vi "Control Scaling.vi"(1 "Position to go":T1={"X"=FALSE, "Target X (um)"=1000.0, "Current X (um)"=1000.0, "Scaling X"=0, "Y"=FALSE, "Target Y (um)"=0.0, "Current Y (um)"=0.0, "Scaling Y"=0, "Z"=FALSE, "Target Z (um)"=0.0, "Current Z (um)"=0.0, "Scaling Z"=0} {"Current X (um)" step=1.0; "Scaling Z" items=["X", "Z", "None"]; "Scaling Y" items=["X", "Z", "None"]; "Scaling X" items=["X", "Z", "None"]; "Target X (um)" step=1.0}) -> (0 "Position to go out":T2)   [LabVIEW 2014]
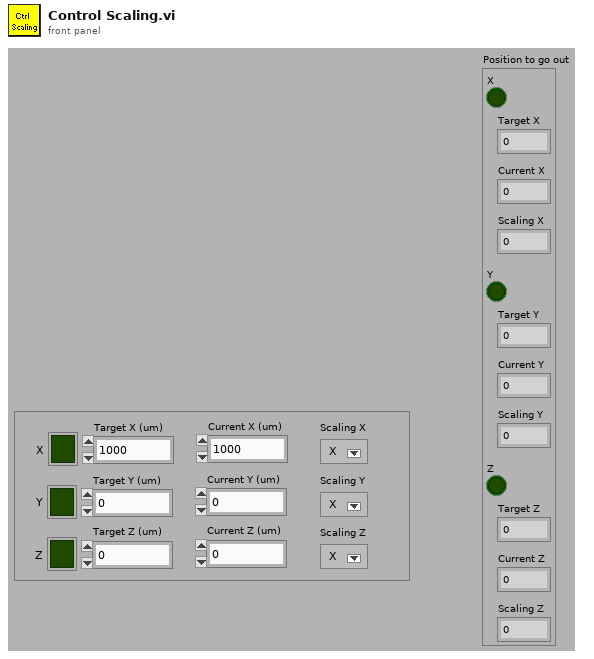
[diagram p1: front panel]
types:
  T1 = cluster{"X":bool, "Target X (um)":dbl, "Current X (um)":dbl, "Scaling X":u16, "Y":bool, "Target Y (um)":dbl, "Current Y (um)":dbl, "Scaling Y":u16, "Z":bool, "Target Z (um)":dbl, "Current Z (um)":dbl, "Scaling Z":u16}
  T2 = cluster{"X":bool, "Target X ":dbl, "Current X":dbl, "Scaling X":u16, "Y":bool, "Target Y":dbl, "Current Y":dbl, "Scaling Y":u16, "Z":bool, "Target Z":dbl, "Current Z":dbl, "Scaling Z":u16}
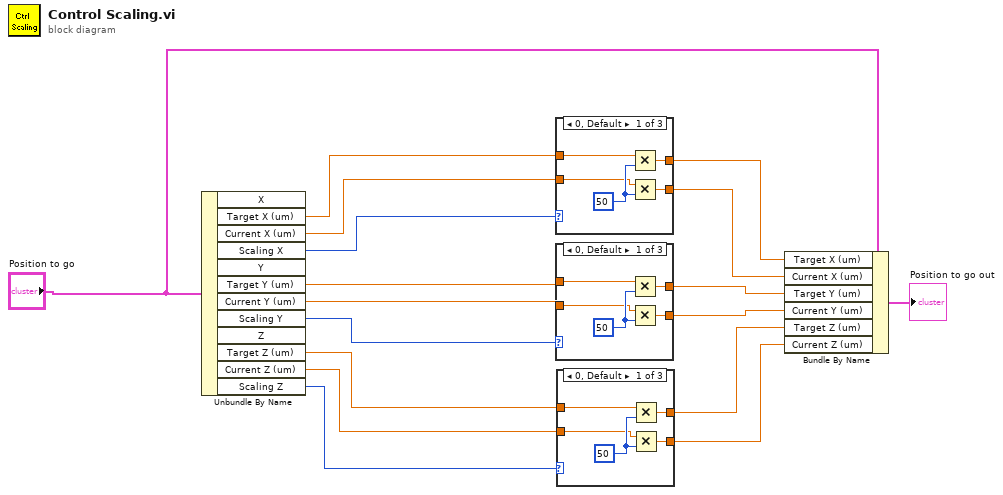
[diagram p0: block diagram]
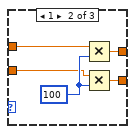
[diagram p2: hidden frame]
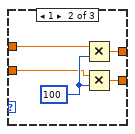
[diagram p4: hidden frame]
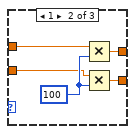
[diagram p6: hidden frame]
diagram:
  n1 = Unbundle By Name("Position to go") -> ("Target X (um)"=w17:dbl, "Current X (um)"=w16:dbl, "Scaling X"=w15:u16, "Target Y (um)"=w14:dbl, "Current Y (um)"=w13:dbl, "Scaling Y"=w12:u16, "Target Z (um)"=w10:dbl, "Current Z (um)"=w9:dbl, "Scaling Z"=w11:u16)  [unwired: 3 out]
  n2 = case shown="0, Default" w15 {
    tunnel: [w22 w25 w28] -> w7
    tunnel: w17 -> [w20 w24 w29]
    tunnel: w16 -> [w19 w23 w28]
    tunnel: [w18 w26 w29] -> w8
    frame 0, Default {
      w21 = 50
      n3 = Multiply(x=w20, y=w21) -> (x*y=w18:dbl)
      n4 = Multiply(x=w19, y=w21) -> (x*y=w22:dbl)
    }
    frame 1 {
      w27 = 100
      n5 = Multiply(x=w24, y=w27) -> (x*y=w26:dbl)
      n6 = Multiply(x=w23, y=w27) -> (x*y=w25:dbl)
    }
    frame 2 {
    }
  }
  n7 = case shown="0, Default" w12 {
    tunnel: [w34 w37 w40] -> w5
    tunnel: w14 -> [w32 w36 w41]
    tunnel: w13 -> [w31 w35 w40]
    tunnel: [w30 w38 w41] -> w6
    frame 0, Default {
      w33 = 50
      n8 = Multiply(x=w32, y=w33) -> (x*y=w30:dbl)
      n9 = Multiply(x=w31, y=w33) -> (x*y=w34:dbl)
    }
    frame 1 {
      w39 = 100
      n10 = Multiply(x=w36, y=w39) -> (x*y=w38:dbl)
      n11 = Multiply(x=w35, y=w39) -> (x*y=w37:dbl)
    }
    frame 2 {
    }
  }
  n12 = case shown="0, Default" w11 {
    tunnel: [w46 w49 w52] -> w3
    tunnel: w10 -> [w44 w48 w53]
    tunnel: w9 -> [w43 w47 w52]
    tunnel: [w42 w50 w53] -> w4
    frame 0, Default {
      w45 = 50
      n13 = Multiply(x=w44, y=w45) -> (x*y=w42:dbl)
      n14 = Multiply(x=w43, y=w45) -> (x*y=w46:dbl)
    }
    frame 1 {
      w51 = 100
      n15 = Multiply(x=w48, y=w51) -> (x*y=w50:dbl)
      n16 = Multiply(x=w47, y=w51) -> (x*y=w49:dbl)
    }
    frame 2 {
    }
  }
  n17 = Bundle By Name(cluster="Position to go", "Target X (um)"=w8, "Current X (um)"=w7, "Target Y (um)"=w6, "Current Y (um)"=w5, "Target Z (um)"=w4, "Current Z (um)"=w3) -> (→"Position to go out":T1)
